vi "testScriptingAddLoopbackUDP.vi"(8 "error in (no error)":errorcluster, 11 "TestCase in":refnum<class "Scripting.lvclass">) -> (0 "error out":errorcluster, 3 "TestCase out":refnum<class "Scripting.lvclass">)   [LabVIEW 2017, in "Scripting.lvclass"]
uses:
  Scripting.lvclass
  <vilib>/addons/_JKI Toolkits/VI Tester/TestCase.llb/TestCase.lvclass
  <vilib>/NI Veristand/Execution/Workspace/NI_VS Workspace ExecutionAPI.lvlib
  b55b5565-dc34-4e51-bcfa-5a6cba25043e.vi
  df0c3853-f0b6-44a9-ad36-32614d313efc.vi
  <vilib>/NI Veristand/Execution/Workspace/NI VeriStand - Set Multiple Channel Values.vi
  <vilib>/NI Veristand/Execution/Workspace/NI VeriStand - Get Multiple Channel Values.vi
  C:/Git/niveristand-custom-device-testing-tools/VeriStandTestCase/VeriStandTestCase.lvclass
  C:/Program Files (x86)/National Instruments/LabVIEW 2017/vi.lib/addons/_JKI Toolkits/VI Tester/TestCase.llb/TestCase.lvclass
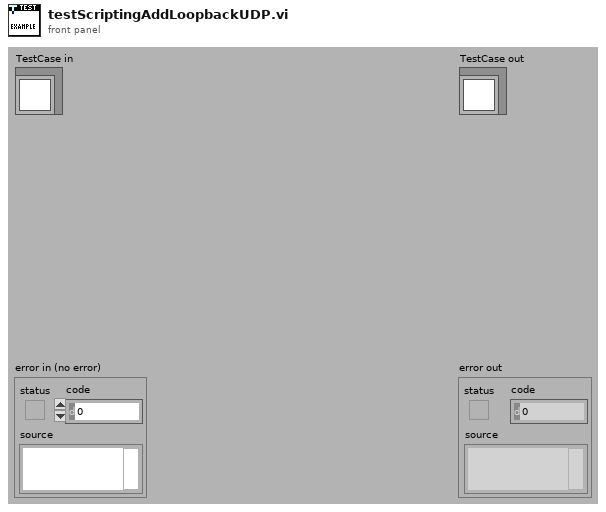
[diagram p1: front panel]
types:
  T1 = typedef "NI_VS Workspace ExecutionAPI.lvlib/WorkspaceAPI.ctl" = refnum<k24>
  T2 = typedef "NI_VS Workspace ExecutionAPI.lvlib/NodeInfo.ctl" = cluster{"Name":string, "FullPath":string, "Type":string, "IsChannel":bool, "Channel":cluster{"Unit":string, "Readable":bool, "Writable":bool, "Faultable":bool, "Scalable":bool, "RowDim":u32, "ColumnDim":u32, "Value Table Names":string[], "Value Table Values":dbl[]}, "IsWaveform":bool, "Waveform":cluster{"DataType":T3}}
  T3 = typedef "NI_VS Workspace ExecutionAPI.lvlib/Waveform Data Type.ctl" = enum16{"Double", "ComplexDouble"}
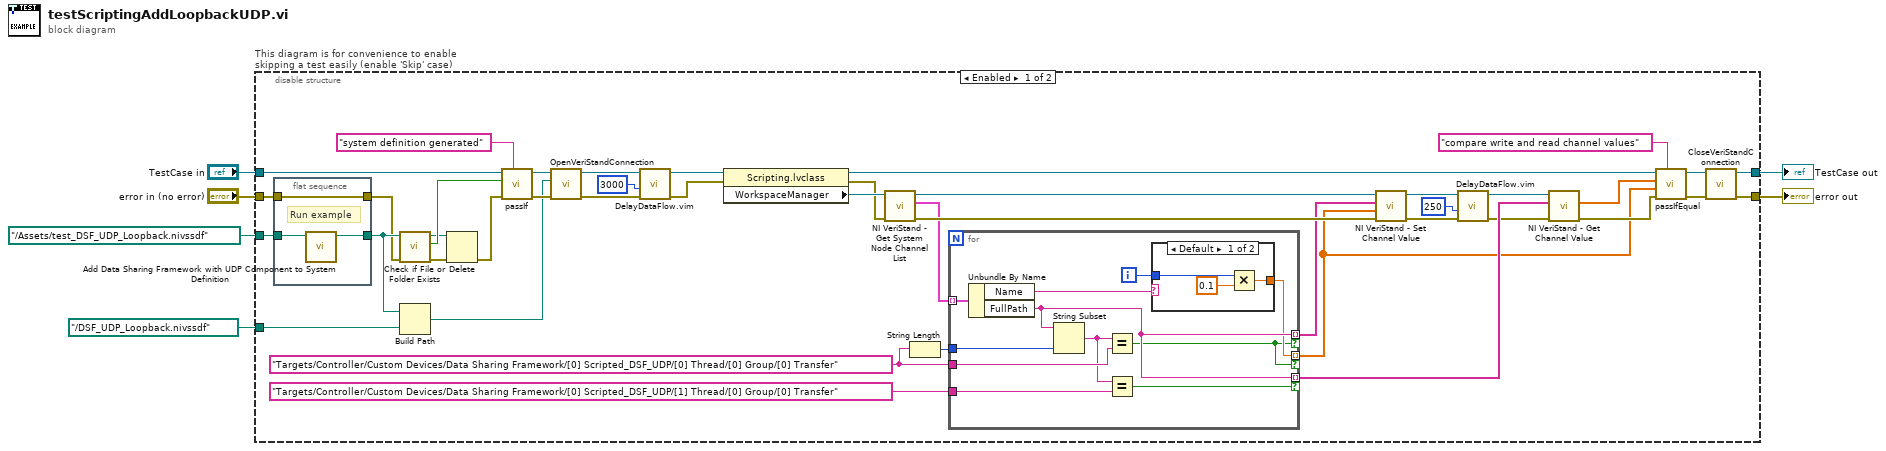
[diagram p0: block diagram]
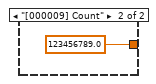
[diagram p2: hidden frame]
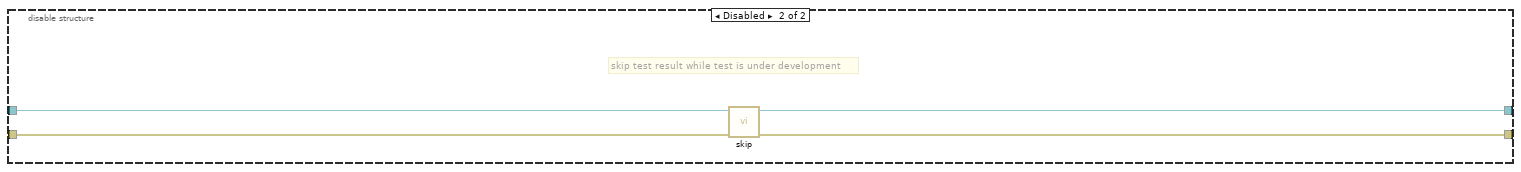
[diagram p3: hidden frame]
diagram:
  n1 = disable-structure "This diagram is for convenience to enable skipping a test easily (enable 'Skip' case)" shown="Enabled" {
    disable-tunnel: "TestCase in" -> [w28 w69]
    disable-tunnel: [w41 w67] -> w3
    disable-tunnel: [w39 w68] -> w4
    disable-tunnel: "error in (no error)" -> [w38 w66]
    disable-tunnel: path "../Assets/test_DSF_UDP_Loopback.nivssdf" ("Output System Definition File") -> [w33 _]
    disable-tunnel: path "../DSF_UDP_Loopback.nivssdf" ("Created System Definition File") -> [w32 _]
    frame Enabled {
      w20 = "Targets/Controller/Custom Devices/Data Sharing Framework/[0] Scripted_DSF_UDP/[0] Thread/[0] Group/[0] Transfer" ("FullPath")
      n2 = flat-sequence {
        tunnel: w38 -> [w65]
        tunnel: [w65] -> w26
        tunnel: [w64] -> w31
        tunnel: w33 -> [w63]
        frame #0 {
          # "Run example"
          n3 = call "Add Data Sharing Framework with UDP Component to System Definition.vi"("Output System Definition File"=w63) -> ("Created System Definition File"=w64:path)  [unwired: 10 in]
        }
      }
      n4 = call <vilib>:"Check if File or Folder Exists.vi"("error in (no error)"=w26, "path"=w31) -> ("error out"=w25:errorcluster, "file or folder exists?"=w30:bool, "dup path"=w23:path)  [unwired: 7 in]
      n5 = Build Path(base path=w31, name or relative path=w32) -> (appended path=w22:path)
      n6 = Delete(path (use dialog)=w23, error in=w25) -> (error out=w24:errorcluster)  [unwired: 3 in, 2 out]
      n7 = call-dynamic "passIf.vi"("custom report message (\"\")"="system definition generated" ("custom report message (\"\")"), "error in (no error)"=w24, "pass"=w30, "TestCase in"=w28) -> ("error out"=w29:errorcluster, "TestCase out"=w27:refnum<class "Scripting.lvclass">)  [unwired: 6 in]
      n8 = call-dynamic "OpenVeriStandConnection.vi"("error in (no error)"=w29, "System Definition File"=w22, "VeriStand Test Case in"=w27) -> ("error out"=w44:errorcluster, "VeriStand Test Case out"=w47:refnum<class "Scripting.lvclass">)  [unwired: 6 in, 1 out]
      n9 = call "DelayDataFlow.vim"("value in"=w44, "milliseconds to wait"=u32 3000) -> ("value out"=w43:errorcluster)  [unwired: 2 in, 1 out]
      n10 = property class="Scripting.lvclass"(reference=w47, error in=w43) -> (reference out=w46:refnum<class "Scripting.lvclass">, error out=w35:errorcluster, "WorkspaceManager"=w37:T1)
      n11 = call <vilib>:"NI VeriStand - Get System Node Channel List.vi"("error in (no error)"=w35, "WorkspaceManager in"=w37) -> ("error out"=w34:errorcluster, "Channels"=w19:T2[], "WorkspaceManager out"=w36:T1)  [unwired: 7 in]
      n12 = String Length(string=w20) -> (length=w21:i32)
      n13 = for {
        tunnel: w19 -> [w58] mode=indexing
        tunnel: w21 -> [w57]
        tunnel: w20 -> [w56]
        tunnel: [w51] -> w18 mode=indexing if=w48
        tunnel: "Targets/Controller/Custom Devices/Data Sharing Framework/[0] Scripted_DSF_UDP/[1] Thread/[0] Group/[0] Transfer" ("FullPath") -> [w55]
        tunnel: [w51] -> w16 mode=indexing if=w53
        tunnel: [w49] -> w8 mode=indexing if=w48
        i -> [w50]
        n14 = Unbundle By Name(w58) -> ("Name"=w52:string, "FullPath"=w51:string)
        n15 = String Subset(string=w51, length (rest)=w57) -> (substring=w54:string)  [unwired: 1 in]
        n16 = Equal?(x=w54, y=w56) -> (x = y?=w48:bool)
        n17 = Equal?(x=w54, y=w55) -> (x = y?=w53:bool)
        n18 = case shown="Default" w52 {
          tunnel: w50 -> [w61 _]
          tunnel: [w59 123456789.0] -> w49
          frame Default {
            n19 = Multiply(x=w61, y=0.1) -> (x*y=w59:dbl)
          }
          frame "[000009] Count" {
          }
        }
      }
      n20 = call-poly <vilib>:"NI VeriStand - Set Channel Value.vi"("error in (no error)"=w34, "Values"=w8, "Channels"=w18, "WorkspaceManager in"=w36) -> ("error out"=w15:errorcluster, "WorkspaceManager out"=w13:T1)  [unwired: 6 in]
      n21 = call "DelayDataFlow.vim"("value in"=w15, "milliseconds to wait"=u32 250) -> ("value out"=w14:errorcluster)  [unwired: 2 in, 1 out]
      n22 = call-poly <vilib>:"NI VeriStand - Get Channel Value.vi"("error in (no error)"=w14, "Channels"=w16, "WorkspaceManager in"=w13) -> ("error out"=w12:errorcluster, "Values"=w11:dbl[])  [unwired: 6 in, 1 out]
      n23 = call-dynamic "passIfEqual.vi"("custom report message (\"\")"="compare write and read channel values" ("custom report message (\"\")"), "error in (no error)"=w12, "y"=w8, "x"=w11, "TestCase in"=w46) -> ("error out"=w40:errorcluster, "TestCase out"=w42:refnum<class "Scripting.lvclass">)  [unwired: 5 in]
      n24 = call-dynamic "CloseVeriStandConnection.vi"("error in (no error)"=w40, "VeriStand Test Case in"=w42) -> ("error out"=w39:errorcluster, "VeriStand Test Case out"=w41:refnum<class "Scripting.lvclass">)  [unwired: 8 in]
    }
    frame Disabled {
      # "skip test result while test is under development"
      n25 = call <vilib>:"skip.vi"("error in (no error)"=w66, "TestCase in"=w69) -> ("error out"=w68:errorcluster, "TestCase out"=w67:refnum<class "Scripting.lvclass">)  [unwired: 8 in]
    }
  }
  "error out" <- w4
  "TestCase out" <- w3
